vi "Actor Core.vi"(8 "error in":errorcluster, 11 "Debugger in":refnum<class "Debugger.lvclass">) -> (0 "error out":errorcluster, 3 "Actor out":refnum<class "Actor.lvclass">)   [LabVIEW 2019, in "Debugger.lvlib" / "Debugger.lvclass"]
doc: "The user interface for this panel.\n\n----\nPlease see the following web address for additional documentation and tutorial information:\nhttp://www.mooregoodideas.com/mgi-panel-manager/\n\nAuthor: Derek Trepanier\n\nCopyright (c) 2018, Moore Good Ideas, Inc.\n\nAll rights reserved.\n\nRedistribution and use in source and binary forms, with or without modification, are permitted provided that the following conditions are met:\n\n * Redistributions of source code must retain the above copyright notice, this list of conditions and the following disclaimer.\n * Redistributions in binary form must reproduce the above copyright notice, this list of conditions and the following disclaimer in the documentation and/or other materials provided with the distribution.\n * Neither the name of Moore Good Ideas, Inc. nor the names of its contributors may be used to endorse or promote products derived from this software without specific prior written permission.\n\nTHIS SOFTWARE IS PROVIDED BY THE COPYRIGHT HOLDERS AND CONTRIBUTORS \"AS IS\" AND ANY EXPRESS OR IMPLIED WARRANTIES, INCLUDING, BUT NOT LIMITED TO, THE IMPLIED WARRANTIES OF MERCHANTABILITY AND FITNESS FOR A PARTICULAR PURPOSE ARE DISCLAIMED. IN NO EVENT SHALL THE COPYRIGHT OWNER OR CONTRIBUTORS BE LIABLE FOR ANY DIRECT, INDIRECT, INCIDENTAL, SPECIAL, EXEMPLARY, OR CONSEQUENTIAL DAMAGES (INCLUDING, BUT NOT LIMITED TO, PROCUREMENT OF SUBSTITUTE GOODS OR SERVICES; LOSS OF USE, DATA, OR PROFITS; OR BUSINESS INTERRUPTION) HOWEVER CAUSED AND ON ANY THEORY OF LIABILITY, WHETHER IN CONTRACT, STRICT LIABILITY, OR TORT (INCLUDING NEGLIGENCE OR OTHERWISE) ARISING IN ANY WAY OUT OF THE USE OF THIS SOFTWARE, EVEN IF ADVISED OF THE POSSIBILITY OF SUCH DAMAGE."
uses:
  Library/Debugger.lvclass
  C:/Users/Public/Documents/Development/builds/Engine/Engine.lvlibp/Project/Engine.lvclass
  builds/Engine/Actor Framework.lvlibp/1abvi3w/vi.lib/ActorFramework/Actor/Actor.lvclass
  builds/Engine/Engine.lvlibp/Accessors/Write VI_Ref.vi
  builds/Base Software/Panels/Left Panel.lvlibp/Project/Left.lvclass
  builds/Engine/Engine.lvlibp/Project/Engine.lvclass
panel:
  in  "Supply name":string
  in  "Supply State":bool
  in  "Error":bool
  in  "Warning":bool
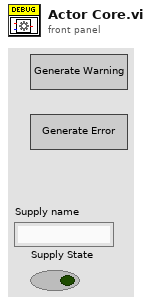
[diagram p1: front panel]
types:
  T1 = cluster{"Pnl Actor":refnum<event-registration>, "Event Registration Refnum":refnum<event-registration>}
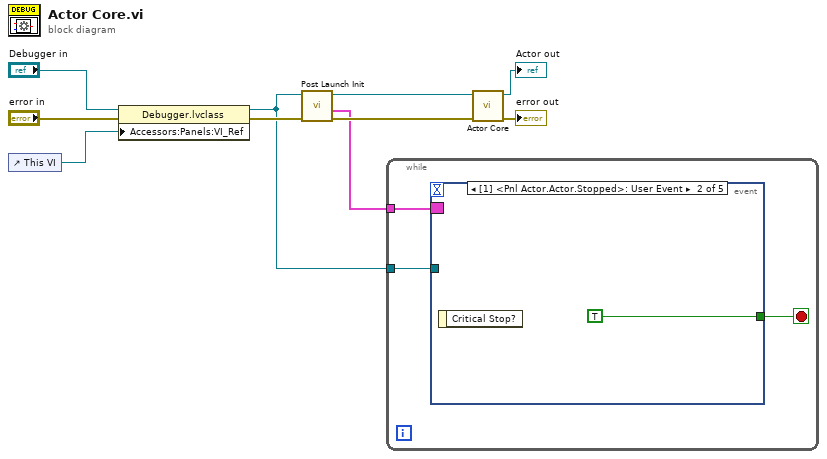
[diagram p0: block diagram]
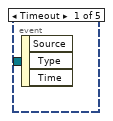
[diagram p2: hidden frame]
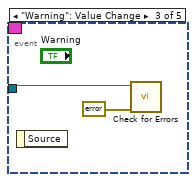
[diagram p3: hidden frame]
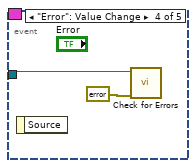
[diagram p4: hidden frame]
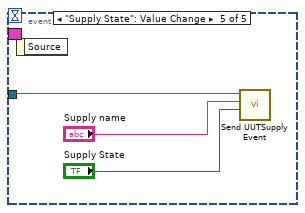
[diagram p5: hidden frame]
diagram:
  n1 = control-ref of="This VI"() -> (w6:refnum<vi>)
  n2 = property class="Debugger.lvclass"(reference="Debugger in", error in="error in", "Accessors:Panels:VI_Ref"=w6) -> (reference out=w4:refnum<class "Debugger.lvclass">, error out=w5:errorcluster)
  n3 = call "Post Launch Init.vi"("error in"=w5, "Debugger in"=w4) -> ("error out"=w2:errorcluster, "output cluster"=w1:T1, "Debugger out"=w3:refnum<class "Debugger.lvclass">)  [unwired: 7 in]
  n4 = while {
    tunnel: w4 -> [w12]
    tunnel: w1 -> [w11]
    stop <- w13 stop-if-true
    n5 = event shown="[1] <Pnl Actor.Actor.Stopped>: User Event" {
      selector: w11 -> [_ _ _ _ _]
      dyn-events: _ -> [_ _ _ _ _]
      timeout: _ -> [_ _ _ _ _]
      tunnel: [_ TRUE _ _ _] -> w13
      tunnel: w12 -> [_ _ w16 w18 w21]
      event Timeout {
        n6 = event-data() -> ()  [unwired: 1 in, 3 out]
      }
      event User Event {
        n7 = event-data() -> ()  [unwired: 1 in, 1 out]
      }
      event "Warning": Value Change {
        n8 = event-data() -> ()  [unwired: 1 in, 1 out]
        n9 = call "Check for Errors.vi"("error in"=errorcluster {"status"=FALSE, "code"=8000, "source"="Warning Generated"}, "Engine in"=w16) -> ()  [unwired: 8 in, 2 out]
      }
      event "Error": Value Change {
        n10 = event-data() -> ()  [unwired: 1 in, 1 out]
        n11 = call "Check for Errors.vi"("error in"=errorcluster {"status"=TRUE, "code"=8001, "source"="Error Generated"}, "Engine in"=w18) -> ()  [unwired: 8 in, 2 out]
      }
      event "Supply State": Value Change {
        n12 = event-data() -> ()  [unwired: 1 in, 1 out]
        n13 = call "Send UUTSupply Event.vi"("Output"="Supply State", "Supply"="Supply name", "Engine in"=w21) -> ()  [unwired: 7 in, 2 out]
      }
    }
  }
  n14 = call-parent "Actor Core.vi"("error in"=w2, "Left in"=w3) -> ("error out"=→"error out":errorcluster, "Actor out"=→"Actor out":refnum<class "Actor.lvclass">)  [unwired: 8 in]
